vi "DAQNavi Write (Digital 1D Wfm NChan NSamp).vi"(8 "error in (no error)":errorcluster, 9 "timeout":dbl=10.0, 10 "data":digitalwaveform[](array[waveform]), 11 "task in":i32) -> (0 "error out":errorcluster, 2 "number of samples written per channel":u32, 3 "task out":i32)   [LabVIEW 2020]
uses:
  <vilib>/Waveform/DWDTOps.llb/DWDT Digital to Binary U8.vi
  DAQNavi_LV.dll
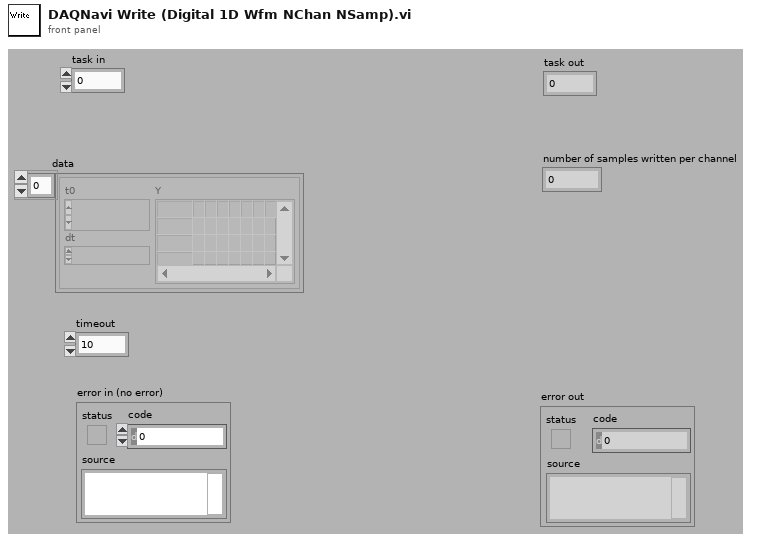
[diagram p1: front panel]
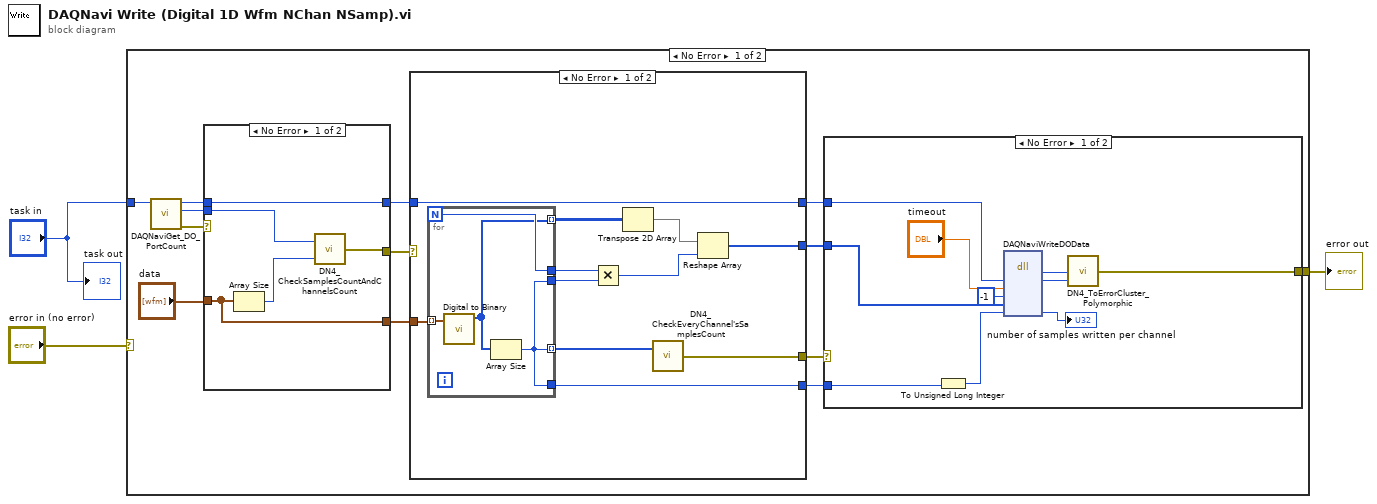
[diagram p0: block diagram]
diagram:
  n1 = case shown="No Error" "error in (no error)" {
    selector: "error in (no error)" -> [_ w53]
    tunnel: [w12 w53] -> w2
    tunnel: "task in" -> [w13 _]
    frame No Error {
      n2 = call "DAQNaviGet_DO_PortCount.vi"("task in"=w13) -> ("error out"=w16:errorcluster, "port count"=w15:i32, "task out"=w14:i32)  [unwired: 1 in, 7 out]
      n3 = case shown="No Error" w16 {
        selector: w16 -> [_ w41]
        tunnel: w15 -> [w36 _]
        tunnel: [w34 w41] -> w11
        tunnel: [w38 w40] -> w8
        tunnel: w14 -> [w38 w40]
        tunnel: "data" -> [w37 w39]
        tunnel: [w37 w39] -> w10
        frame No Error {
          n4 = Array Size(array=w37) -> (size(s)=w35:i32)
          n5 = call "DN4_CheckSamplesCountAndChannelsCount.vi"("samples count"=w35, "channel count"=w36) -> ("error out"=w34:errorcluster)
        }
        frame Error {
        }
      }
      n6 = case shown="No Error" w11 {
        selector: w11 -> [_ w33]
        tunnel: w10 -> [w27 _]
        tunnel: [w18 w33] -> w9
        tunnel: [w23 w32] -> w7
        tunnel: w8 -> [w23 w32]
        tunnel: [w22 _] -> w6
        tunnel: [w17 _] -> w5
        frame No Error {
          n7 = for {
            N -> [w31]
            tunnel: w27 -> [w29] mode=indexing
            tunnel: [w30] -> w26 mode=indexing
            tunnel: [w28] -> w24 mode=indexing
            tunnel: [w30] -> w21
            tunnel: [w31] -> w20
            tunnel: [w30] -> w17
            n8 = call-poly <vilib>:"Digital to Binary.vi"("digital waveform"=w29) -> ("binary array"=w28:u8[])  [unwired: 1 in, 9 out]
            n9 = Array Size(array=w28) -> (size(s)=w30:i32)
          }
          n10 = Multiply(x=w20, y=w21) -> (x*y=w19:i32)
          n11 = Transpose 2D Array(2D array=w24) -> (transposed array=w25:u8[][])
          n12 = call "DN4_CheckEveryChannel'sSamplesCount.vi"("samples count"=w26) -> ("error out"=w18:errorcluster)  [unwired: 1 in]
          n13 = Reshape Array(w25, w19) -> (w22:u8[])
        }
        frame Error {
        }
      }
      n14 = case shown="No Error" w9 {
        selector: w9 -> [_ w52]
        tunnel: [w51 w52] -> w12
        tunnel: w7 -> [w47 _]
        tunnel: w6 -> [w44 _]
        tunnel: w5 -> [w46 _]
        frame No Error {
          n15 = To Unsigned Long Integer(number=w46) -> (unsigned 32bit integer=w45:u32)
          n16 = dll-call lib="DAQNavi_LV.dll" fn="DAQNaviWriteDOData"("taskID"=w47, "timeout"="timeout", "portBit"=-1, "portData"=w44, "samples"=w45) -> ("return type"=w48:i32, "taskID"=w43:i32, "samples"=→"number of samples written per channel":u32)  [unwired: 6 in, 2 out]
          n17 = call "DN4_ToErrorCluster_Polymorphic.vi"("task id"=w43, "error code"=w48) -> ("error out"=w51:errorcluster)  [unwired: 3 out]
        }
        frame Error {
        }
      }
    }
    frame Error {
    }
  }
  "error out" <- w2
  "task out" <- "task in"
